vi "SetValue.vi"(8 "error in":errorcluster, 10 "Value":i32, 11 "NonNegativeInt in":refnum<class "NonNegativeInt.lvclass">) -> (0 "error out":errorcluster, 3 "NonNegativeInt out":refnum<class "NonNegativeInt.lvclass">)   [LabVIEW 2021, in "ProligentXMLGenerator.lvlib" / "NonNegativeInt.lvclass"]
uses:
  NonNegativeInt.lvclass
  NonNegativeInt.lvclass/NonNegativeInt.ctl
  Int/Int.lvclass
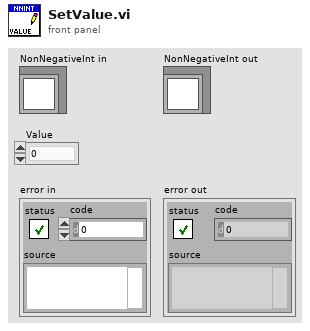
[diagram p1: front panel]
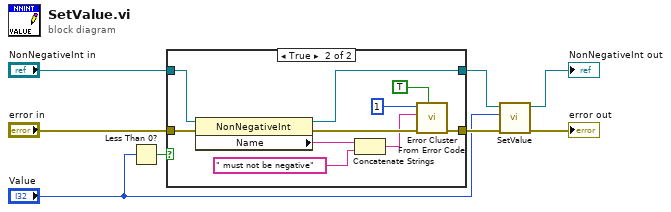
[diagram p0: block diagram]
diagram:
  n1 = Less Than 0?(x="Value") -> (x < 0?=w3:bool)
  n2 = case shown="True" w3 {
    tunnel: "error in" -> [w10 w14]
    tunnel: [w10 w20] -> w4
    tunnel: [w9 w12] -> w2
    tunnel: "NonNegativeInt in" -> [w9 w15]
    frame False {
    }
    frame True {
      n3 = property on="Property Node" class="NonNegativeInt"(reference=w15, error in=w14) -> (reference out=w12:refnum<class "NonNegativeInt.lvclass">, error out=w13:errorcluster, "Name"=w16:string)
      n4 = Concatenate Strings(w16, " must not be negative" ("string")) -> (w11:string)
      n5 = call <vilib>:"Error Cluster From Error Code.vi"("show call chain? (False)"=TRUE, "error in (no error)"=w13, "error message (\"\")"=w11, "error code (0)"=1) -> ("error out"=w20:errorcluster)  [unwired: 5 in]
    }
  }
  n6 = call-parent "SetValue.vi"("error in"=w4, "Value"="Value", "Int in"=w2) -> ("error out"=→"error out":errorcluster, "Int out"=→"NonNegativeInt out":refnum<class "NonNegativeInt.lvclass">)  [unwired: 7 in]
